vi "Untitled 1.vi"   [LabVIEW 2013]
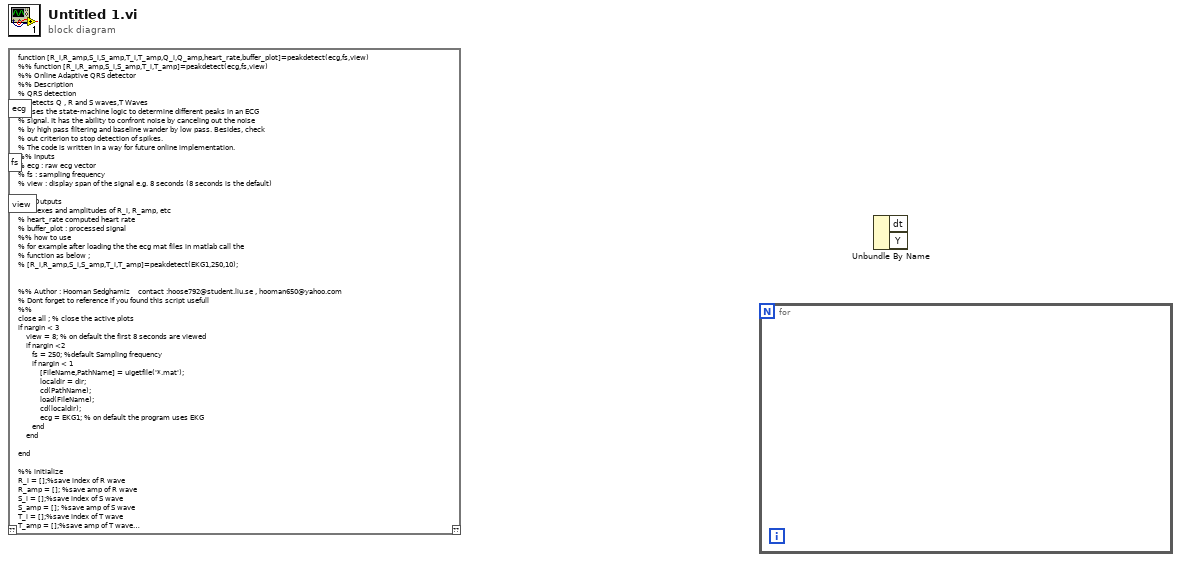
[diagram p0: block diagram]
diagram:
  n1 = script code="function [R_i,R_amp,S_i,S_amp,T_i,T_amp,Q_i,Q_amp,heart_rate,buffer_plot]=peakdetect(ecg,fs,view)\n%% function [R_i,R_amp,S_i,S_amp,T_i,T_amp]=peakdetect(ecg,fs,view)\n%% Online Adaptive QRS detector\n%% Description\n% QRS detection\n% Detects Q , R and S waves,T Waves\n% Uses the state-machine logic to determine different peaks in an ECG\n% signal. It has the ability to confront noise by canceling out the noise\n% by high pass filtering and baseline wander by low pass. Besides, check\n% out criterion to stop detection of spikes.\n% The code is written in a way for future online implementation.\n%% Inputs\n% ecg : raw ecg vector\n% fs : sampling frequency\n% view : display span of the signal e.g. 8 seconds (8 seconds is the default)\n\n%% Outputs\n% indexes and amplitudes of R_i, R_amp, etc\n% heart_rate computed heart rate\n% buffer_plot : processed signal\n%% how to use\n% for example after loading the the ecg mat files in matlab call the\n% function as below ;\n% [R_i,R_amp,S_i,S_amp,T_i,T_amp]=peakdetect(EKG1,250,10);\n\n\n%% Author : Hooman Sedghamiz    contact :hoose792@student.liu.se , hooman650@yahoo.com\n% Dont forget to reference if you found this script usefull\n%%\nclose all ; % close the active plots\nif nargin < 3\n    view = 8; % on default the first 8 seconds are viewed\n    if nargin <2\n       fs = 250; %default Sampling frequency\n       if nargin < 1\n           [FileName,PathName] = uigetfile('*.mat');\n           localdir = dir;\n           cd(PathName);\n           load(FileName);\n           cd(localdir);\n           ecg = EKG1; % on default the program uses EKG\n       end\n    end\n    \nend\n\n%% initialize\nR_i = [];%save index of R wave\nR_amp = []; %save amp of R wave\nS_i = [];%save index of S wave\nS_amp = []; %save amp of S wave\nT_i = [];%save index of T wave\nT_amp = [];%save amp of T wave\nthres_p =[]; %for plotting adaptive threshold\nbuffer_plot =[];\nbuffer_long=[]; % buffer for online processing\nstate = 0 ; % determines the state of the machine in the algorithm\nc = 0; % counter to determine that the state-machine doesnt get stock in T wave detection wave\nT_on = 0; % counter showing for how many samples the signal stayed above T wave threshold\nT_on1=0; % counter to make sure its the real onset of T wave\nS_on = 0; % counter to make sure its the real onset of S wave\nsleep = 0; % counter that avoids the detection of several R waves in a short time\nS_amp1 = []; % buffer to set the adaptive T wave onset\nbuffer_base=[]; %buffer to determine online adaptive mean of the signal\ndum = 0; %counter for detecting the exact R wave\nwindow = round(fs/25); % averaging window size\nweight = 1.8; %initial value of the weigth\nco = 0; % T wave counter to come out of state after a certain time\nthres2_p = []; %T wave threshold indices\nthres_p_i = []; %to save indices of main thres\nS_amp1_i = []; %to save indices of S thres\nthres2_p_i = []; %to save indices of T threshold\nQ_i = []; % vectors to store Q wave\nQ_amp =[]; %vectors to store Q wave\n%% preprocess\necg = ecg (:); % make sure its a vector\necg_raw =ecg; %take the raw signal for plotting later\ntime_scale = length(ecg_raw)/fs; % total time;\n%Noise cancelation(Filtering)\nf1=0.5; %cuttoff low frequency to get rid of baseline wander\nf2=45; %cuttoff frequency to discard high frequency noise\nWn=[f1 f2]*2/fs; % cutt off based on fs\nN = 3; % order of 3 less processing\n[a,b] = butter(N,Wn); %bandpass filtering\necg = filtfilt(a,b,ecg);\n\n%% define two buffers\n\nbuffer_mean=mean(abs(ecg(1:2*fs)-mean(ecg(1:2*fs)))); % adaptive threshold DC corrected (baseline removed)\nbuffer_T = mean(ecg(1:2*fs));%second adaptive threshold to be used for T wave detection\n%% start online inference (Assuming the signal is being acquired online)\nfor i = 1 : length(ecg)\n    \nbuffer_long = [buffer_long ecg(i)] ; % save the upcoming new samples\nbuffer_base = [buffer_base ecg(i)] ; % save the baseline samples\n\n%% Renew the mean and adapt it to the signal after 1 second of processing\nif length(buffer_base) >= 2*fs\n    buffer_mean = mean(abs(buffer_base(1:2*fs)-mean(buffer_base(1:2*fs))));\n    buffer_T = mean(buffer_base(1:2*fs));\n    buffer_base =[];\nend\n\n%% smooth the signal by taking the average of 15 samples and add the new upcoming samples\n  if length(buffer_long)>= window % take a window with length 15 samples for averaging\n      mean_online = mean(buffer_long);  % take the mean\n      buffer_plot =[buffer_plot mean_online]; % save the processed signal\n      \n      \n    %% Enter state 1(putative R wave) as soon as that the mean exceeds the double time of threshold  \n    if state == 0  \n     if length(buffer_plot) >= 3   %added to handle bugg for now\n      if mean_online > buffer_mean*weight && buffer_plot(i-1-window) > buffer_plot(i-window)    %2.4*buffer_mean   \n          state = 1; % entered R peak detection mode\n          currentmax = buffer_plot(i-1-window);\n          ind = i-1-window;\n          thres_p = [thres_p buffer_mean*weight];\n          thres_p_i = [thres_p_i ind];\n      else     \n          state = 0;\n      end\n     end\n    end\n    \n    %% Locate the R wave location by finding the highest local maxima\n      if state == 1 % look for the highest peak\n          \n            if  currentmax > buffer_plot(i-window)\n                dum = dum + 1;\n                if dum > 4 \n                R_i = [R_i ind];%save index\n                R_amp = [R_amp buffer_plot(ind)]; %save index\n                % Locate Q wave\n                [Q_tamp Q_ti] = min(buffer_plot(ind-round(0.040*fs):(ind)));\n                Q_ti = ind-round(0.040*fs) + Q_ti -1;\n                Q_i = [Q_i Q_ti];\n                Q_amp = [Q_amp Q_tamp];\n                \n                \n                if length(R_amp) > 8\n                weight = 0.30*mean(R_amp(end-7:end)); %calculate the 35% of the last 8 R waves\n                weight = weight/buffer_mean;\n                end\n                state = 2; % enter S detection mode state 2\n                dum = 0;\n                end\n            else\n                dum = 0;\n                state = 0;\n            end \n            \n      end\n      \n    %% check weather the signal drops below the threshold to look for S wave\n      if state == 2 \n        if  mean_online <= buffer_mean     % check the threshold\n             state = 3;   %enter S detection           \n        end\n      end\n      \n      %% Enter S wave detection state3 (S detection)\n          if state == 3\n            co = co + 1; \n            \n          if co < round(0.200*fs)\n            if buffer_plot(i-window-1) <= buffer_plot(i-window) % see when the slope changes\n             S_on = S_on + 1; % set a counter to see if its a real change or just noise\n             if S_on >= round(0.0120*fs)\n             S_i = [S_i i-window-4];%save index of S wave\n             S_amp = [S_amp buffer_plot(i-window-4)];%save index\n             S_amp1 = [S_amp1  buffer_plot(i-window-4)]; %ecg(i-4)\n             S_amp1_i = [S_amp1_i ind]; %index of S_amp1_i\n             state = 4; % enter T detection mode\n             S_on = 0;\n             co = 0;\n             end\n            end\n          else\n              state = 4;\n              co = 0;\n          end\n          end\n      \n       %% enter state 4 possible T wave detection\n       if state == 4    \n         if mean_online < buffer_mean % see if the signal drops below mean \n           state = 6; % confirm\n         end\n       end\n       %% Enter state 6 which is T wave possible detection\n       if state ==6   \n         c = c + 1; % set a counter to exit the state if no T wave detected after 0.3 second\n         if c <= 0.7*fs  \n             % set a double threshold based on the last detected S wave and\n             % baseline of the signal and look for T wave in between these\n             % two threshold\n             thres2 = ((abs(abs(buffer_T)-abs(S_amp1(end))))*3/4 + S_amp1(end)); \n             thres2_p =[thres2_p thres2];\n             thres2_p_i =[thres2_p_i ind];\n             if mean_online > thres2\n              T_on = T_on +1; % make sure it stays on for at least 3 samples\n              if T_on >= round(0.0120*fs)\n               if buffer_plot(i-window-1)>= buffer_plot(i-window)\n                   T_on1 = T_on1+1; % make sure its a real slope change\n                  if T_on1 > round(0.0320*fs) \n                   T_i = [T_i i-window-11];%save index of T wave\n                   T_amp = [T_amp  buffer_plot(i-window-11)];%save index\n                   state = 5; % enter sleep mode\n                   T_on = 0;\n                   T_on1 = 0;\n                  end\n                                      \n               end\n              end\n             end\n             \n            \n          \n         else\n             state= 5; % enter Sleep mode\n         end\n         \n       end  \n      \n        \n       %% this state is for avoiding the detection of a highly variate noise or another peak\n       % this avoids detection of two peaks R waves less than half a second\n       if state==5\n           sleep =sleep+c+1;\n           c = 0;\n           if sleep/fs >= 0.400\n               state = 0;\n               sleep = 0;%look for the next peak\n           end  \n       end\n      \n      % update the online buffer by removing the oldest sample\n      buffer_long(1)=[];\n      \n      \n  end\n  \nend\n\n%% conditions\nR_R = diff(R_i); % calculate the distance between each R wave\nheart_rate=length(R_i)/(time_scale/60); % calculate heart rate\nmsgbox(strcat('Heart-rate is = ',mat2str(heart_rate)));\n% compute the min max R-R wave\nmax_R_interval = max(R_R);\nmin_R_interval = min(R_R);\n% detect arythmia if there is any irregularity\n% if (max_R_interval/fs)-(min_R_interval/fs) > 0.16\n%     msgbox('Irregular Rhythm','Arrythmia Detected');\n% end\n\n\n%% plottings \ntime = 1/fs:1/fs:view;\nR = find(R_i <= view*fs); % determine the length for plotting vectors\n%S = find(S_i <= view*fs); % determine the length for plotting vectors\nT = find(T_i <= view*fs); % determine the length for plotting vectors\n%Q = find(Q_i <= view*fs); % determine the length for plotting vectors\nL1 = find(thres_p_i <= view*fs);\nL2 = find(S_amp1_i <= view*fs);\nL3 = find(thres2_p_i <= view*fs);\nif view*fs > length(buffer_plot)\nax(1) = subplot(211);plot(time(1:length(buffer_plot)),buffer_plot(1:end));   \nelse\nax(1) = subplot(211);plot(time,buffer_plot(1:(view*fs)));\nend\nhold on,scatter(R_i(1:R(end))./fs,R_amp(1:R(end)),'r');\n%hold on,scatter(S_i(1:S(end))./fs,S_amp(1:S(end)),'g');\nhold on,scatter(T_i(1:T(end))./fs,T_amp(1:T(end)),'k');\n%hold on,scatter(Q_i(1:Q(end))./fs,Q_amp(1:Q(end)),'m');\nhold on,plot(thres_p_i(1:L1(end))./fs,thres_p(1:L1(end)),'LineStyle','-.','color','r',...\n    'LineWidth',2.5);\nhold on,plot(S_amp1_i(1:L2(end))./fs,S_amp1(1:L2(end)),'LineStyle','--','color','c',...\n    'LineWidth',2.5);\nhold on,plot(thres2_p_i(1:L3(end))./fs,thres2_p(1:L3(end)),'-k','LineWidth',2);\nlegend('Raw ECG Signal','R wave','T wave','Latest S wave','T wave adaptive threshold threshold','Location','NorthOutside','Orientation','horizontal'); \nxlabel('Time(sec)'),ylabel('V');\naxis tight; title('Zoom in to see both signal details overlaied');title('Filtered, smoothed and processed signal');\nax(2) =subplot(212);plot(time,ecg_raw(1:(view*fs)));title('Raw ECG')\nxlabel('Time(sec)'),ylabel('V');\nlegend(); \nlinkaxes(ax,'x');\nzoom on;"() -> ()  [unwired: 4 in, 1 out]
  n2 = for {
  }
  n3 = Unbundle By Name() -> ()  [unwired: 1 in, 2 out]
